vi "Close SystemLink Connection.vi"(0 "SystemLink connection in":T1, 11 "error in (no error)":errorcluster) -> (15 "error out":errorcluster)   [LabVIEW 2017, in "SystemLink_States_API.lvlib"]
doc: "Closes the HTTP handle and connection to the SystemLink server (even if there is an incoming error on the error in input)."
uses:
  SystemLink_States_API.lvlib
  _support/systemlink repo.ctl
  <vilib>/httpClient/ClientHandle.ctl
  <vilib>/httpClient/LabVIEWHTTPClient.lvlib
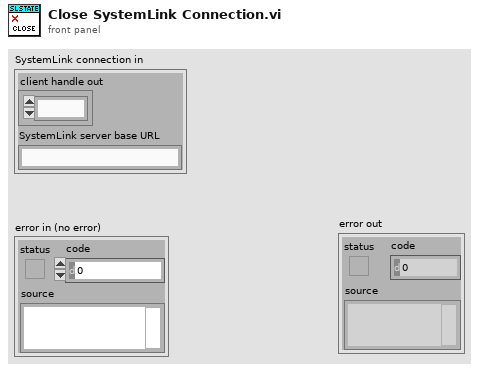
[diagram p1: front panel]
types:
  T1 = typedef "SystemLink_States_API.lvlib/systemlink repo.ctl" = cluster{"client handle out":T2, "SystemLink server base URL":string}
  T2 = typedef "LabVIEWHTTPClient.lvlib/ClientHandle.ctl" = refnum<k1>
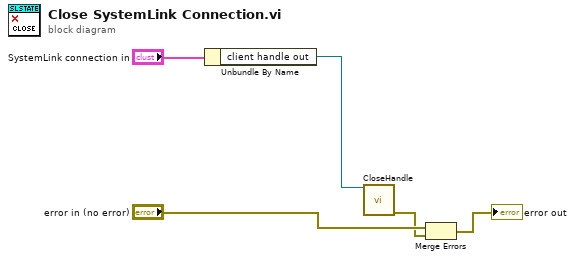
[diagram p0: block diagram]
diagram:
  n1 = Unbundle By Name("SystemLink connection in") -> ("client handle out"=w4:T2)
  n2 = call <vilib>:"CloseHandle.vi"("client handle"=w4) -> ("error out"=w2:errorcluster)  [unwired: 14 in]
  n3 = Merge Errors("error in (no error)", w2) -> (→"error out":errorcluster)
